vi "HMI Normalize.vi"(8 "error in (no error)":errorcluster, 11 "ROV in":refnum<class "ROV Host.lvclass">) -> (0 "error out":errorcluster, 3 "ROV out":refnum<class "ROV Host.lvclass">)   [LabVIEW 2012, in "ROV Host.lvclass"]
uses:
  ROV Host.lvclass
  ROV Host.lvclass/ROV Host.ctl
  <vilib>/Utility/inputDevices.llb/joystickAcquire.vi
panel:
  out "axis info":T1
  out "direction info":T2
  out "button info":T3
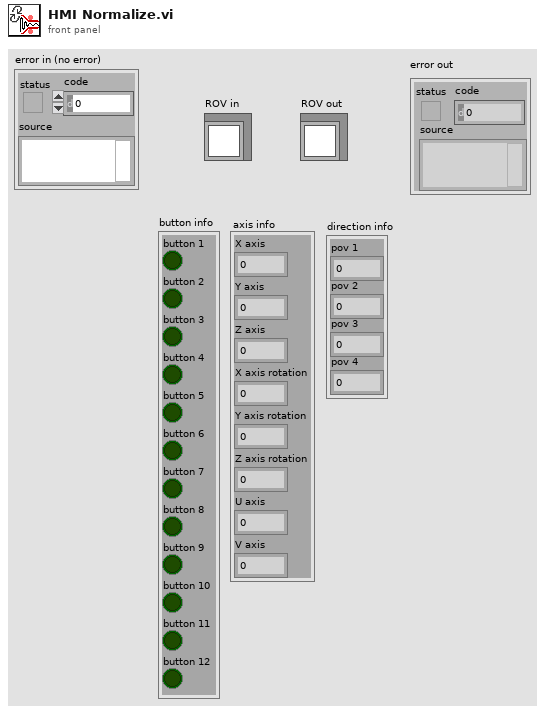
[diagram p1: front panel]
types:
  T1 = cluster{"X axis":i32, "Y axis":i32, "Z axis":i32, "X axis rotation":i32, "Y axis rotation":i32, "Z axis rotation":i32, "U axis":i32, "V axis":i32}
  T2 = cluster{"pov 1":i32, "pov 2":i32, "pov 3":i32, "pov 4":i32}
  T3 = cluster{"button 1":bool, "button 2":bool, "button 3":bool, "button 4":bool, "button 5":bool, "button 6":bool, "button 7":bool, "button 8":bool, "button 9":bool, "button 10":bool, "button 11":bool, "button 12":bool, "button 13":bool, "button 14":bool, "button 15":bool, "button 16":bool, "button 17":bool, "button 18":bool, "button 19":bool, "button 20":bool, "button 21":bool, "button 22":bool, "button 23":bool, "button 24":bool, "button 25":bool, "button 26":bool, "button 27":bool, "button 28":bool, "button 29":bool, "button 30":bool, "button 31":bool, "button 32":bool}
  T4 = typedef "NI_Robotics_Steering Class Types.lvlib/Mecanum Steering Frame.ctl" = refnum<class "NI_Robotics_Mecanum Steering Frame.lvclass">
  T5 = typedef "NI_Robotics_Steering Class Types.lvlib/Differential Steering Frame.ctl" = refnum<class "NI_Robotics_Differential Steering Frame.lvclass">
  T6 = cluster{"mecanum steering frame out":T4, "differential steering frame out":T5}
  T7 = cluster{"device ID":refnum<k1>, "Device Name":string, "axis info":cluster{"X axis":dbl[], "Y axis":dbl[], "Z axis":dbl[], "X axis rotation":dbl[], "Y axis rotation":dbl[], "Z axis rotation":dbl[], "U axis":dbl[], "V axis":dbl[]}}
  T8 = cluster{"button info":cluster{"button 1":bool, "button 2":bool, "button 3":bool, "button 4":bool, "button 5":bool, "button 6":bool, "button 7":bool, "button 8":bool, "button 9":bool, "button 10":bool, "button 11":bool, "button 12":bool, "button 13":bool, "button 14":bool, "button 15":bool, "button 16":bool, "button 17":bool, "button 18":bool, "button 19":bool, "button 20":bool, "button 21":bool, "button 22":bool, "button 23":bool, "button 24":bool, "button 25":bool, "button 26":bool, "button 27":bool, "button 28":bool, "button 29":bool, "button 30":bool, "button 31":bool, "button 32":bool}, "direction info":cluster{"pov 1":i32, "pov 2":i32, "pov 3":i32, "pov 4":i32}, "axis info":cluster{"X axis":i32, "Y axis":i32, "Z axis":i32, "X axis rotation":i32, "Y axis rotation":i32, "Z axis rotation":i32, "U axis":i32, "V axis":i32}}
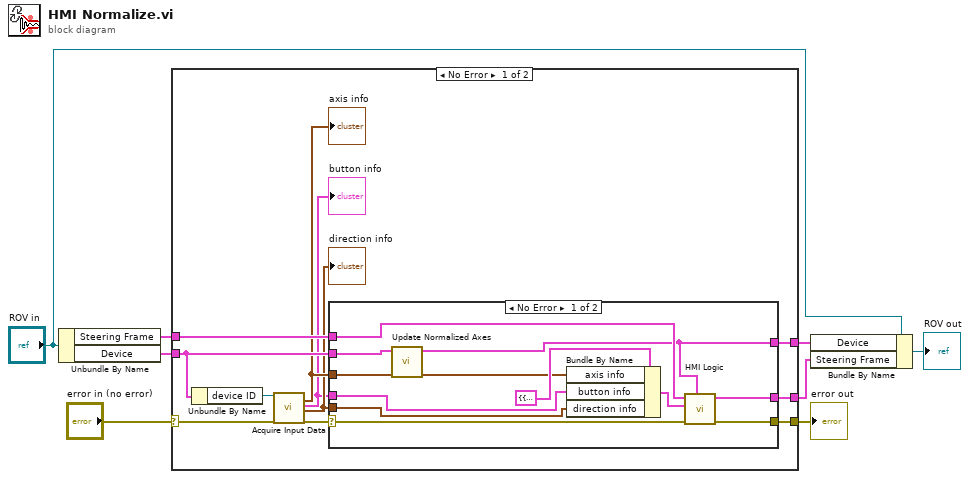
[diagram p0: block diagram]
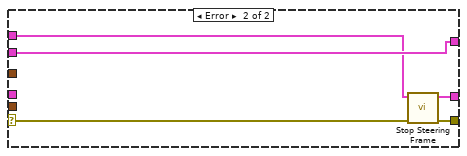
[diagram p2: hidden frame]
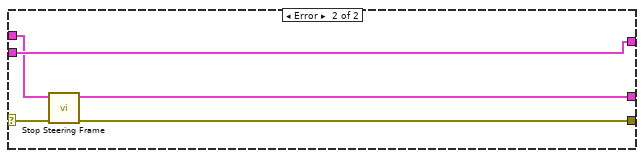
[diagram p3: hidden frame]
diagram:
  n1 = Unbundle By Name("ROV in") -> ("Steering Frame"=w6:T6, "Device"=w5:T7)
  n2 = case shown="No Error" "error in (no error)" {
    selector: "error in (no error)" -> [w14 w39]
    tunnel: [w13 w38] -> w8
    tunnel: w5 -> [w17 w41]
    tunnel: w6 -> [w16 w40]
    tunnel: [w15 w37] -> w2
    tunnel: [w12 w41] -> w1
    frame No Error {
      n3 = Unbundle By Name(w17) -> ("device ID"=w18:refnum<k1>)
      n4 = call-poly <vilib>:"Acquire Input Data.vi"("device ID"=w18, "error in (no error)"=w14) -> ("axis info"=w11:T1, "button info"=w9:T3, "direction info"=w10:T2, "error out"=w19:errorcluster)  [unwired: 13 in, 1 out]
      "axis info" <- w11
      "direction info" <- w10
      "button info" <- w9
      n5 = case shown="No Error" w19 {
        selector: w19 -> [w29 w35]
        tunnel: w11 -> [w31 _]
        tunnel: w17 -> [w30 w36]
        tunnel: w16 -> [w22 w32]
        tunnel: [w27 w33] -> w15
        tunnel: [w28 w34] -> w13
        tunnel: [w21 w36] -> w12
        tunnel: w10 -> [w23 _]
        tunnel: w9 -> [w24 _]
        frame No Error {
          n6 = call "Update Normalized Axes.vi"("axis in"=w31, "Device in"=w30) -> ("axis out"=w25:T1, "Device out"=w21:T7)  [unwired: 8 in]
          n7 = Bundle By Name(cluster=T8 {"button info"={"button 1"=FALSE, "button 2"=FALSE, "button 3"=FALSE, "button 4"=FALSE, "button 5"=FALSE, "button 6"=FALSE, "button 7"=FALSE, "button 8"=FALSE, "button 9"=FALSE, "button 10"=FALSE, "button 11"=FALSE, "button 12"=FALSE, "button 13"=FALSE, "button 14"=FALSE, "button 15"=FALSE, "button 16"=FALSE, "button 17"=FALSE, "button 18"=FALSE, "button 19"=FALSE, "button 20"=FALSE, "button 21"=FALSE, "button 22"=FALSE, "button 23"=FALSE, "button 24"=FALSE, "button 25"=FALSE, "button 26"=FALSE, "button 27"=FALSE, "button 28"=FALSE, "button 29"=FALSE, "button 30"=FALSE, "button 31"=FALSE, "button 32"=FALSE}, "direction info"={"pov 1"=-1, "pov 2"=-1, "pov 3"=-1, "pov 4"=-1}, "axis info"={"X axis"=3832, "Y axis"=898, "Z axis"=0, "X axis rotation"=-443, "Y axis rotation"=465, "Z axis rotation"=0, "U axis"=0, "V axis"=0}} ("HMI"), "axis info"=w25, "button info"=w24, "direction info"=w23) -> (w20:T8)
          n8 = call "HMI Logic.vi"("Device"=w21, "error in (no error)"=w29, "HMI"=w20, "Steering Frame in"=w22) -> ("error out"=w28:errorcluster, "Steering Frame out"=w27:T6)  [unwired: 6 in]
        }
        frame Error {
          n9 = call "Stop Steering Frame.vi"("error in (no error)"=w35, "Steering Frame in"=w32) -> ("error out"=w34:errorcluster, "Steering Frame out"=w33:T6)  [unwired: 8 in]
        }
      }
    }
    frame Error {
      n10 = call "Stop Steering Frame.vi"("error in (no error)"=w39, "Steering Frame in"=w40) -> ("error out"=w38:errorcluster, "Steering Frame out"=w37:T6)  [unwired: 8 in]
    }
  }
  "error out" <- w8
  n11 = Bundle By Name(cluster="ROV in", "Device"=w1, "Steering Frame"=w2) -> (→"ROV out":refnum<class "ROV Host.lvclass">)
